vi "notification_v2.0.vi"() -> ()   [LabVIEW 2025]
doc: "Use this template to build a producer/consumer design pattern with events to produce queue items. Use this design pattern instead of the User Interface Event Handler pattern for user interfaces when you want to execute code asynchronously in response to an event without slowing the user interface responsiveness."
panel:
  in  "Enqueue Element":bool
  in  "stop":bool
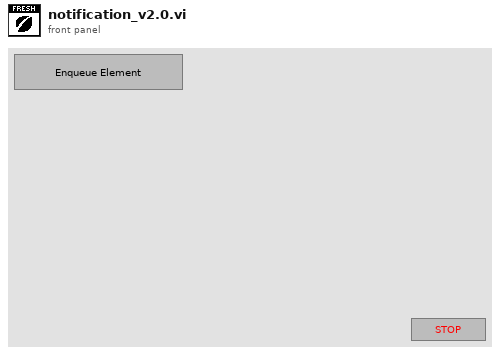
[diagram p1: front panel]
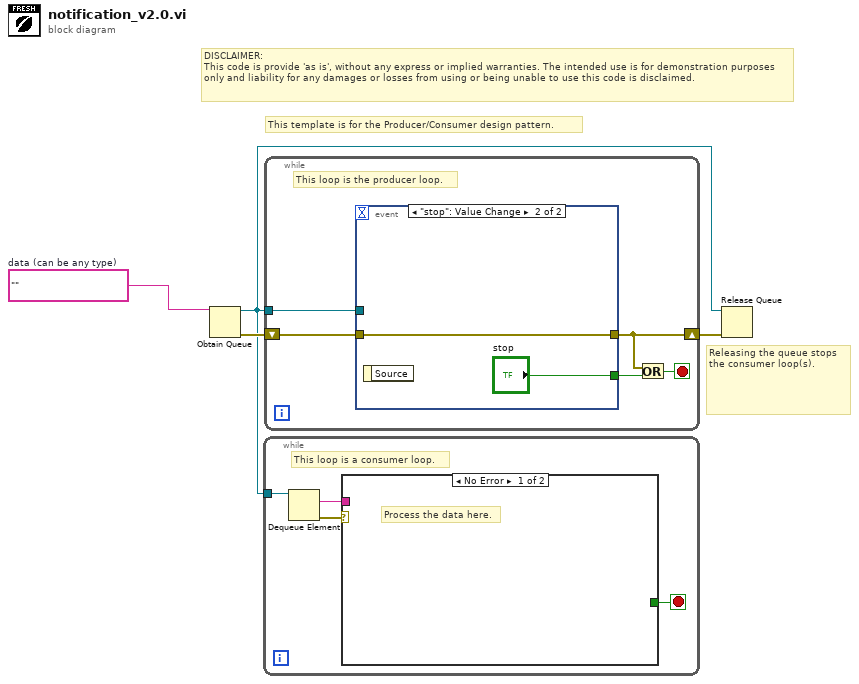
[diagram p0: block diagram]
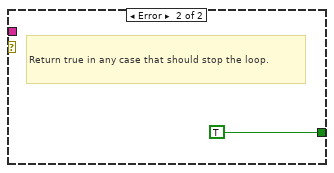
[diagram p2: hidden frame]
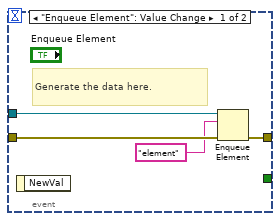
[diagram p3: hidden frame]
diagram:
  w2 = ""  # data (can be any type)
  # "DISCLAIMER:\nThis code is provide 'as is', without any express or implied warranties. The intended use is for demonstration purposes only and liability for any damages or losses from using or being unable to use this code is disclaimed."
  # "Releasing the queue stops the consumer loop(s)."
  # "This template is for the Producer/Consumer design pattern."
  n1 = Obtain Queue(element data type=w2) -> (queue out=w1:refnum<queue>, error out=w4:errorcluster)  [unwired: 4 in, 1 out]
  n2 = while {
    tunnel: w1 -> [w8]
    stop <- w5 stop-if-true
    # "This loop is a consumer loop."
    n3 = Dequeue Element(queue=w8) -> (element=w6:string, error out=w7:errorcluster)  [unwired: 2 in, 2 out]
    n4 = case shown="No Error" w7 {
      tunnel: w6 -> [_ _]
      tunnel: [_ TRUE] -> w5
      frame No Error {
        # "Process the data here."
      }
      frame Error {
        # "Return true in any case that should stop the loop."
      }
    }
  }
  n5 = while {
    shift-right: [w10] -> w3
    shift-left: w4 -> [w13]
    tunnel: w1 -> [w14]
    stop <- w11 stop-if-true
    # "This loop is the producer loop."
    n6 = event shown="[1] \"stop\": Value Change" {
      selector: _ -> [_ _]
      dyn-events: _ -> [_ _]
      timeout: _ -> [_ _]
      tunnel: w14 -> [w18 _]
      tunnel: w13 -> [w17 w19]
      tunnel: [w16 w19] -> w10
      tunnel: [_ "stop"] -> w12
      event "Enqueue Element": Value Change {
        # "Generate the data here."
        n7 = event-data() -> ()  [unwired: 1 in, 1 out]
        n8 = Enqueue Element(queue=w18, element="element", error in (no error)=w17) -> (error out=w16:errorcluster)  [unwired: 1 in, 2 out]
      }
      event "stop": Value Change {
        n9 = event-data() -> ()  [unwired: 1 in, 1 out]
      }
    }
    n10 = Or(x=w10, y=w12) -> (x .or. y?=w11:bool)
  }
  n11 = Release Queue(queue=w1, error in (no error)=w3) -> ()  [unwired: 1 in, 3 out]
